vi "Get List Information.vi"(8 "List Selection":string, 9 "DQMH Scan Info":T2, 10 "References Map":map{string, refnum<vi>}(c390), 11 "Tree Map":T4) -> (1 "Broadcast?":bool, 2 "Vi out":refnum<vi>, 3 "Module type":T1, 5 "DQMH Lib":refnum<vi>)   [LabVIEW 2019, in "Panther Dashboard.lvlib"]
uses:
  Panther Dashboard.lvlib
  <vilib>/National Instruments/Tree Map/Tree Map Data.ctl
  DQMH Modules Info--cluster.ctl
  Module type--enum.ctl
  Project References--cluster.ctl
  <vilib>/National Instruments/Tree Map/Tree Map.lvlib
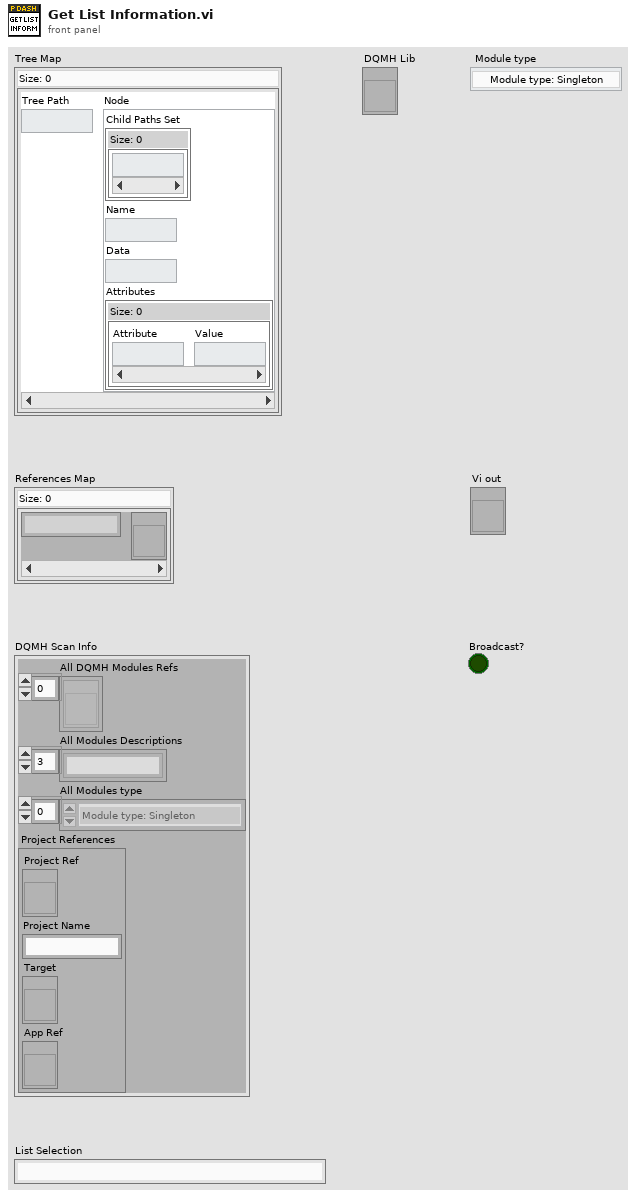
[diagram p1: front panel]
types:
  T1 = typedef "Panther Dashboard.lvlib/Module type--enum.ctl" = enum16{"Module type: Singleton", "Module type: Cloneable"}
  T2 = typedef "Panther Dashboard.lvlib/DQMH Modules Info--cluster.ctl" = cluster{"All DQMH Modules Refs":refnum<vi>[], "All Modules Descriptions":string[], "All Modules type":T1[], "Project References":T3}
  T3 = typedef "Panther Dashboard.lvlib/Project References--cluster.ctl" = cluster{"Project Ref":refnum<vi>, "Project Name":string, "Target":refnum<vi>, "App Ref":refnum<vi>}
  T4 = typedef "Tree Map.lvlib/Tree Map Data.ctl" = map{string, cluster{"Child Paths Set":set{string}, "Name":string, "Data":string, "Attributes":map{string, string}}}
  T5 = cluster{"Child Paths Set":set{string}, "Name":string, "Data":string, "Attributes":map{string, string}}
  T6 = cluster{"Description":string, "VI Description":string}
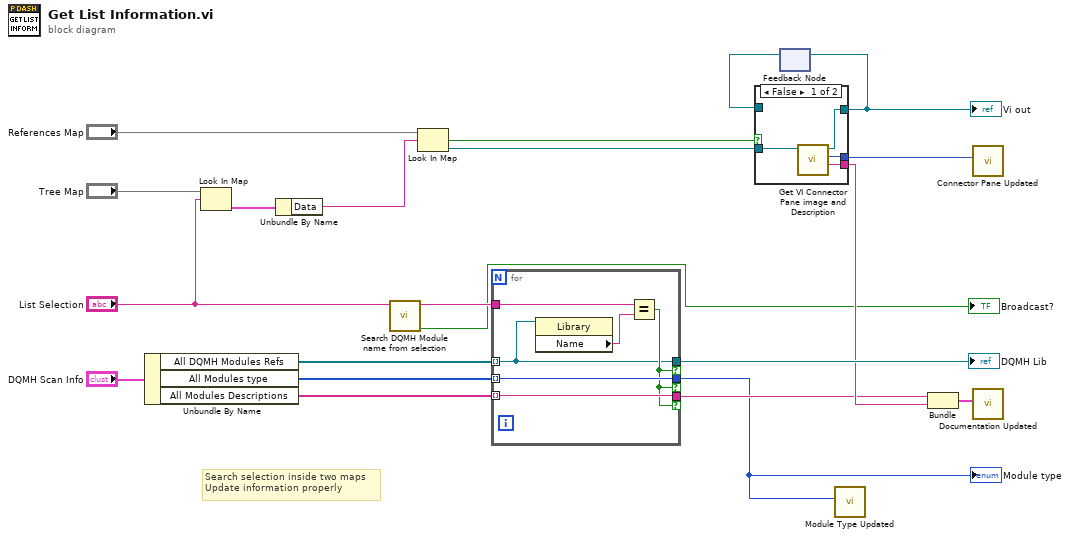
[diagram p0: block diagram]
diagram:
  # "Search selection inside two maps\nUpdate information properly"
  n1 = Unbundle By Name("DQMH Scan Info") -> ("All DQMH Modules Refs"=w13:refnum<vi>[], "All Modules type"=w12:T1[], "All Modules Descriptions"=w11:string[])
  n2 = Look In Map(map="Tree Map", key="List Selection") -> (value=w20:T5)  [unwired: 1 in, 1 out]
  n3 = Unbundle By Name(w20) -> ("Data"=w16:string)
  n4 = call "Search DQMH Module name from selection.vi"("Search Module Name"="List Selection") -> ("Broadcast?"=→"Broadcast?":bool, "Module Name"=w10:string)  [unwired: 9 in]
  n5 = Look In Map(map="References Map", key=w16) -> (key not found?=w17:bool, value=w15:refnum<vi>)  [unwired: 1 in]
  n6 = for {
    tunnel: w13 -> [w23] mode=indexing
    tunnel: w12 -> [w26] mode=indexing
    tunnel: w11 -> [w25] mode=indexing
    tunnel: w10 -> [w27]
    tunnel: [w23] -> w9 if=w24
    tunnel: [w26] -> w1 if=w24
    tunnel: [w25] -> w4 if=w24
    n7 = property class="Library"(reference=w23) -> ("Name"=w22:string)  [unwired: 1 in, 2 out]
    n8 = Equal?(x=w27, y=w22) -> (x = y?=w24:bool)
  }
  "DQMH Lib" <- w9
  "Module type" <- w1
  n9 = feedback #1() -> (w7:refnum<vi>)  [unwired: 1 in]
  n10 = case shown="False" w17 {
    tunnel: w15 -> [w31 _]
    tunnel: [w30 _] -> w3
    tunnel: [w29 w32] -> w8
    tunnel: [w28 _] -> w6
    tunnel: w7 -> [_ w32]
    frame False {
      n11 = call "Get VI Connector Pane image and Description.vi"("VI in"=w31) -> ("VI Description"=w28:string, "VI Connector Pane"=w30:picture, "Vi out"=w29:refnum<vi>)  [unwired: 7 in, 1 out]
    }
    frame True {
    }
  }
  "Vi out" <- w8
  n12 = feedback-in #1(w8) -> ()
  n13 = call "Module Type Updated.vi"("Module Type"=w1) -> ()  [unwired: 10 in, 1 out]
  n14 = Bundle("Description"=w4, "VI Description"=w6) -> (w2:T6)  [unwired: 1 in]
  n15 = call "Connector Pane Updated.vi"("Event Connector Pane"=w3) -> ()  [unwired: 10 in, 1 out]
  n16 = call "Documentation Updated.vi"("Documentation"=w2) -> ()  [unwired: 10 in, 1 out]
